vi "set_active.vi"(8 "error in (no error)":errorcluster, 10 "active (-2=current)":i32=-2, 11 "window in":refnum<class "rywindow.lvclass">) -> (0 "error out":errorcluster, 3 "window out":refnum<class "rywindow.lvclass">)   [LabVIEW 2017, in "rywindow.lvclass"]
uses:
  rywindow.lvclass
  rywindow.lvclass/rywindow.ctl
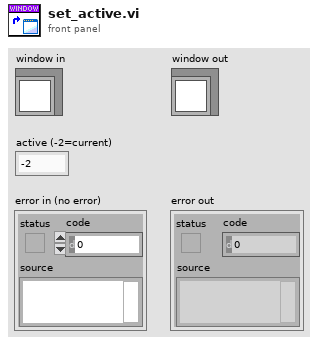
[diagram p1: front panel]
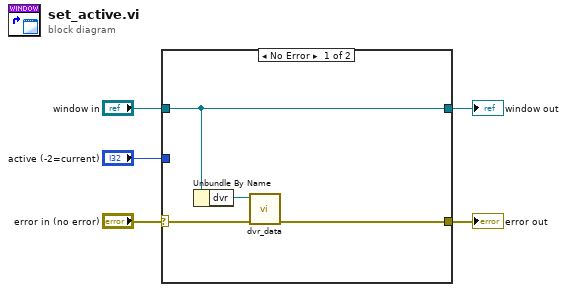
[diagram p0: block diagram]
diagram:
  n1 = case shown="No Error" "error in (no error)" {
    selector: "error in (no error)" -> [w8 w11]
    tunnel: [w7 w11] -> w4
    tunnel: [w9 w10] -> w2
    tunnel: "window in" -> [w9 w10]
    tunnel: "active (-2=current)" -> [_ _]
    frame No Error {
      n2 = Unbundle By Name(w9) -> ("dvr"=w6:refnum<data-value>)
      n3 = call "dvr_data.vi"("error in (no error)"=w8, "dvr"=w6) -> ("error out"=w7:errorcluster)  [unwired: 8 in, 1 out]
    }
    frame Error {
    }
  }
  "error out" <- w4
  "window out" <- w2
